vi "CPP_CalcTubingCorrection.vi"() -> (5 "Plug in titles":string[](array[string]), 7 "Plug in values":string[](array[string]))   [LabVIEW 2013]
uses:
  <vilib>/Analysis/baseanly.llb/Mean (DBL).vi
  Globals/Meas_global.vi
  <vilib>/Analysis/NI_AALBase.lvlib
  <vilib>/Analysis/NI_AALPro.lvlib
panel:
  in  "Tab Control":enum32{"TubingCorrection", "Setup"}(tab)
  in  "RefXducer":i32(ring) items=["Mano (Pref)", "Mano (P15)"]
  in  "TestXducer":i32(ring) items=["Mano (Pref)", "Mano (P15)"]
  out "Time Traces":cluster{dbl, dbl, dbl[][]}(graph)
  out "Spectra":cluster{dbl, "df (Hz)":dbl, dbl[][]}(graph)
  in  "stop":bool
  in  "Pause Button":bool
  in  "Pause(ms)":u32=500
  in  "Coherence Threshold":dbl=0.98
  out "Coefficients Smoothed and Normalized":bool
  in  "Decimate Correction File?":bool=TRUE
  in  "Smooth Correction File?":bool=TRUE
  in  "CorrectionFileDestinationPath":path
  in  "fcut (Hz)":dbl=1000.0
  in  "Cutoff type":string(combo)="Brickwall"
  out "SD(boosted)":dbl format="%.3e"
  out "SD(ref)":dbl format="%.3e"
  out "SD(Boostederror%)":dbl format="%#_3g"
  out "Current Block No":i32
  in  "LowFrequencySmoothingFloor":dbl=3.0
  in  "LowFrequencySmoothingCeiling":dbl=7.0
  in  "ExistingTubingCorrectionFile":path
  in  "Apply Phase Correction?":bool=TRUE
  in  "Save Files?":bool
  in  "Use Existing Correction File?":bool
  out "df (Hz)":dbl format="%.6f"
  in  "Decimation Term":i32=10
  out "OutputString":string
  in  "N Points To Average Either Side":i32=10
  in  "Force Phase 0 Intercept?":bool=TRUE
  out "SD(muted)":dbl format="%.3e"
  out "SD(Mutederror%)":dbl format="%#_3g"
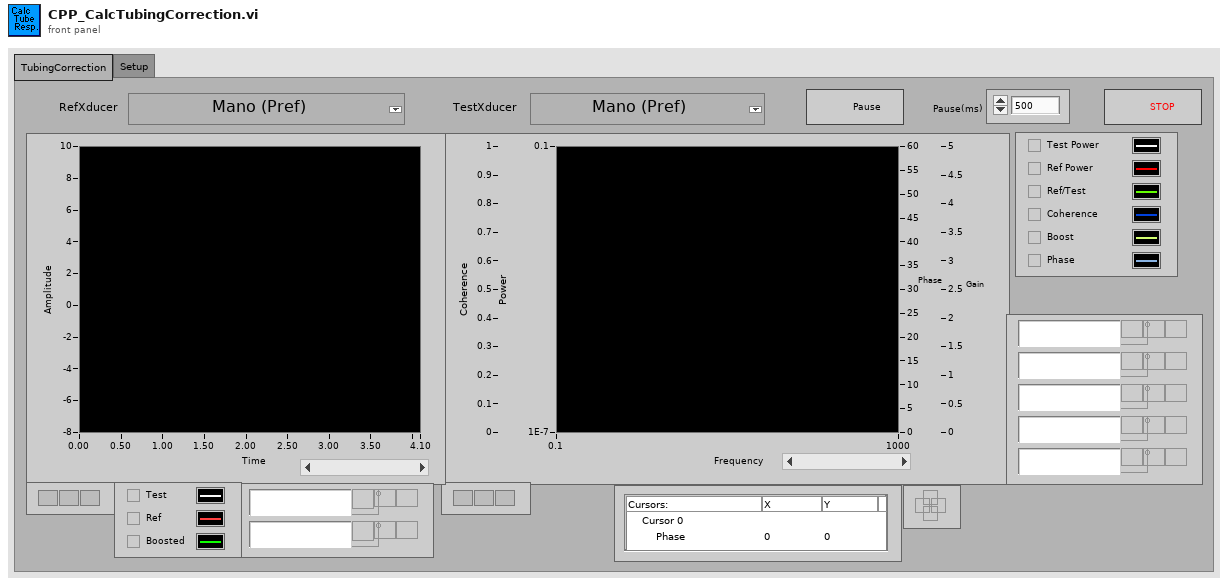
[diagram p1: front panel]
types:
  T1 = typedef "Analysis_info_cluster.ctl" = cluster{"Colour":u32, "Inst type":T2, "Inst name":string, "Symbol":string, "Code name":string, "Extra Info":string, "Inst Array":T3, "Extra Titles":string[], "Extra Values":string[], "U":dbl, "u^2":dbl, "u^3":dbl, "u^4":dbl, "Skew_u":dbl, "Kurt_u":dbl, "Sd Error in Mean":dbl, "% u'/U":dbl, "X":dbl, "Y":dbl, "Z":dbl, "Timescale integral to 25%":dbl, "Sd Error in Variance":dbl, "Calib File":path, "Calib Constants":dbl[], "Output Position":bool, "Full Stats":bool, "Av Sampling Rate":dbl, "Av No of Samples":dbl, "Total Meas Time (s)":dbl, "ADAM Ch Name":string}
  T2 = typedef "Inst_type.ctl" = enum16{"Propeller anemometer", "Raw voltage", "Pressure Transducer", "Pitot-static tube", "Preston tube", "Hot wire", "Cross wire 1", "Cross wire 2", "Generic Linear", "Generic Polynomial", "Generic BackPoly", "Fast FID", "Thermocouple", "Cold wire", "Pulsed Wire", "LDA Vel", "LDA Tran time", "LDA Arr time"}
  T3 = typedef "Instrument_Array.ctl" = enum16{"PWA", "LDA", "Analogue"}
  T4 = typedef "Time_Trace_Cluster.ctl" = cluster{"Weighting":dbl[], "Time (s)":dbl[], "Voltage":dbl[], "Eng Values":dbl[]}
  T5 = enum16{"open", "replace", "create", "open or create", "replace or create", "replace or create with confirmation"}
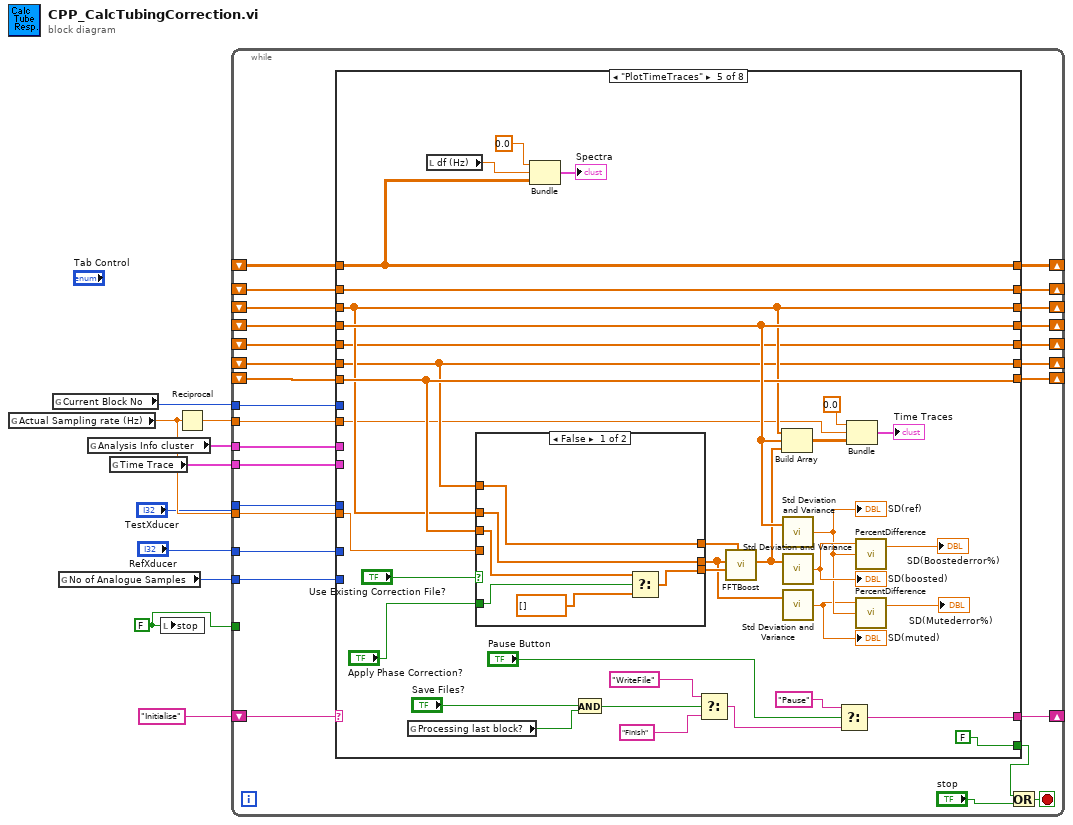
[diagram p0: block diagram]
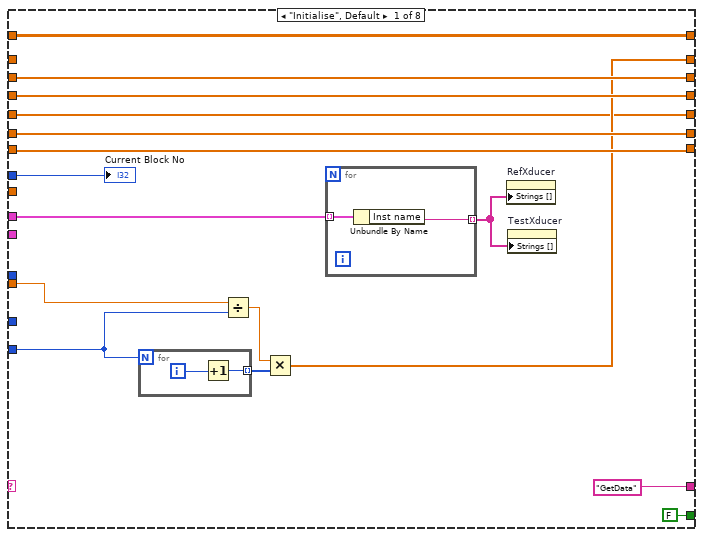
[diagram p2: hidden frame]
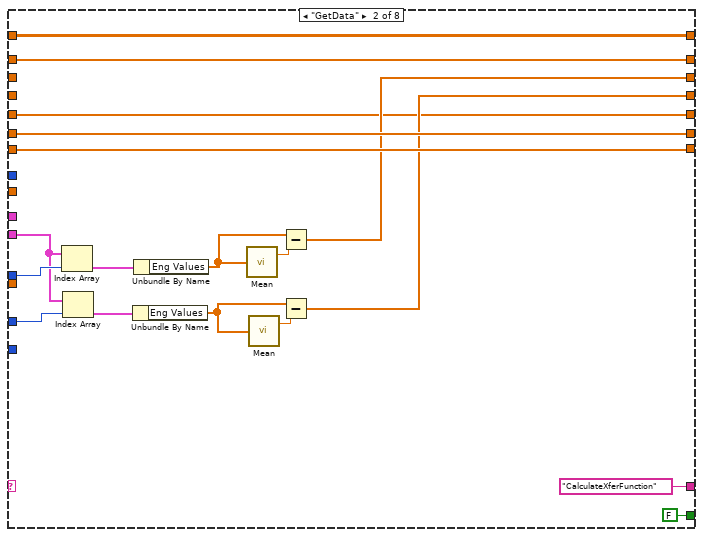
[diagram p3: hidden frame]
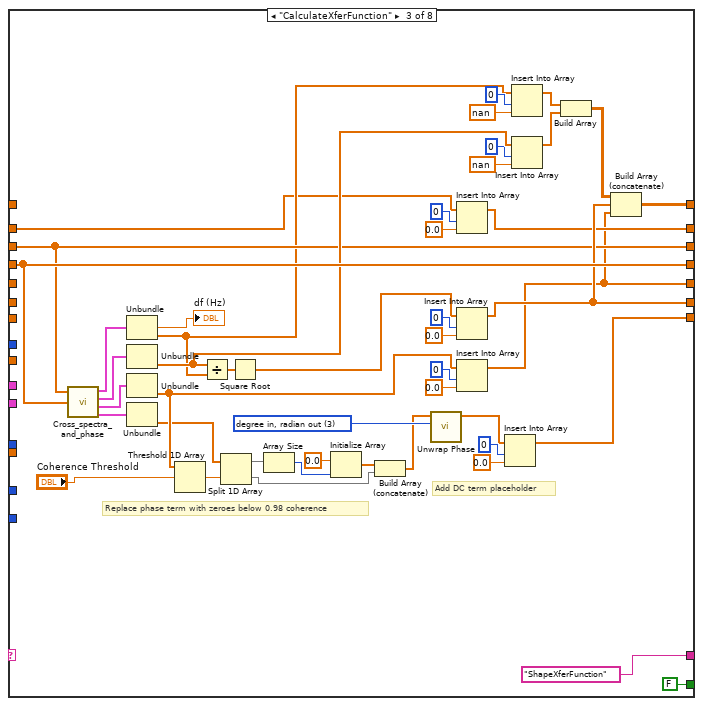
[diagram p4: hidden frame]
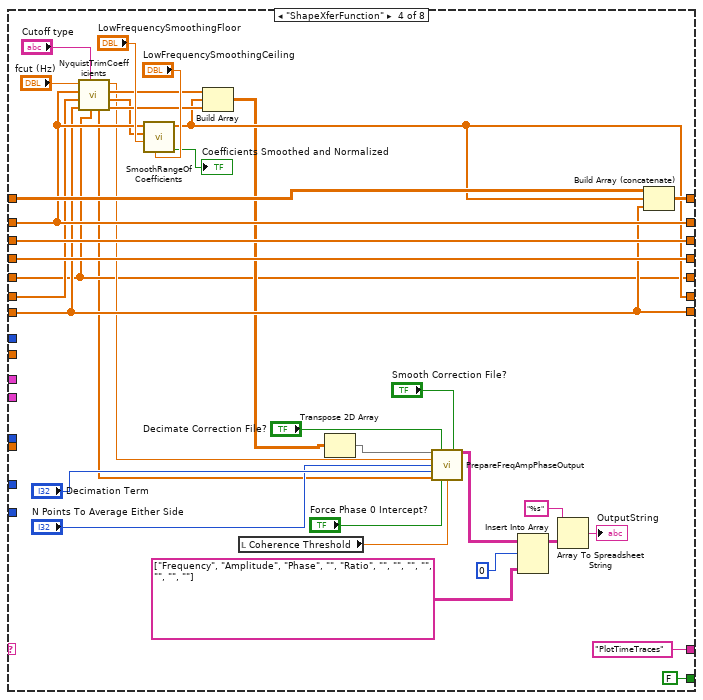
[diagram p5: hidden frame]
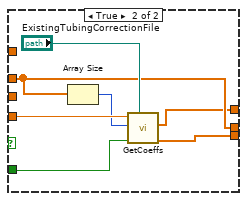
[diagram p6: hidden frame]
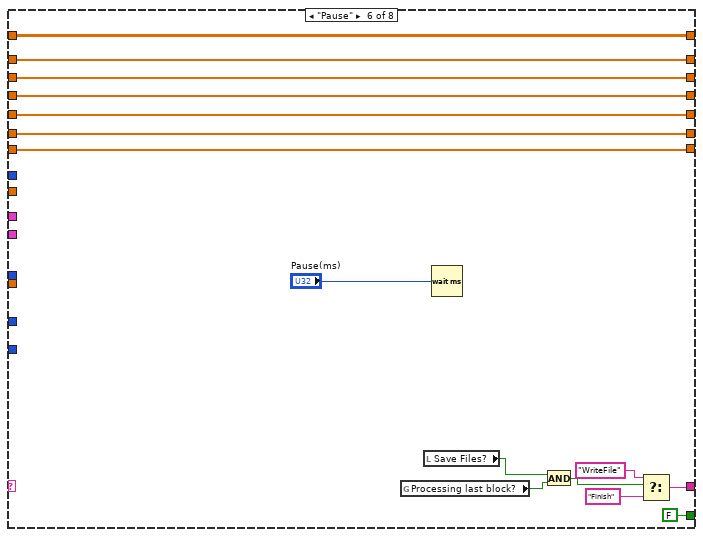
[diagram p7: hidden frame]
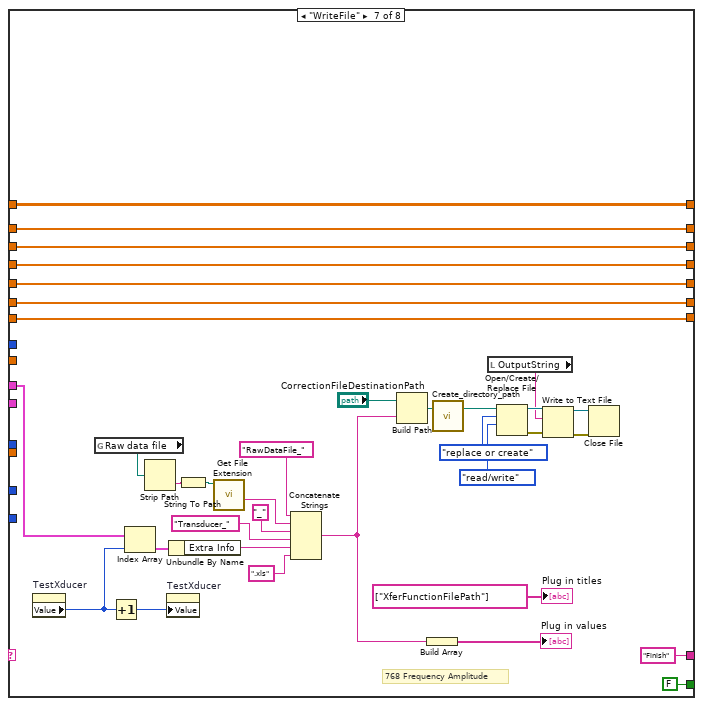
[diagram p8: hidden frame]
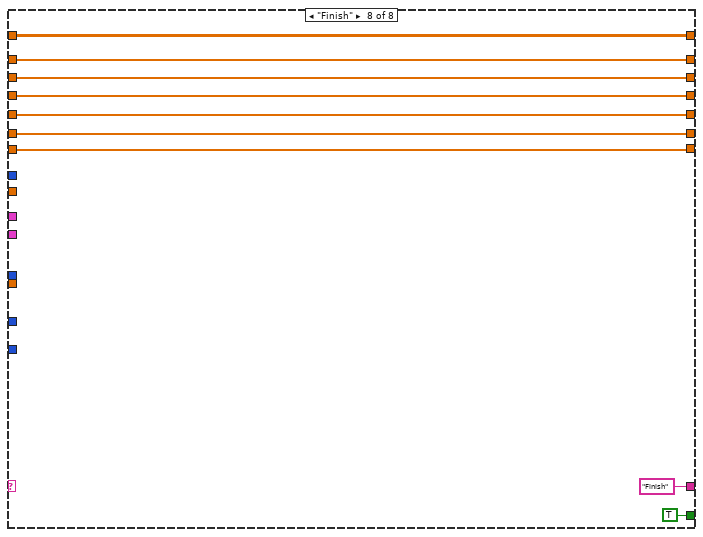
[diagram p9: hidden frame]
diagram:
  w9 = FALSE ("stop")
  n1 = global read "Meas_global.vi" "Actual Sampling rate (Hz)"() -> (w3:dbl)
  n2 = global read "Meas_global.vi" "Current Block No"() -> (w7:i32)
  n3 = global read "Meas_global.vi" "No of Analogue Samples"() -> (w2:i32)
  n4 = global read "Meas_global.vi" "Analysis Info cluster"() -> (w6:T1[])
  n5 = global read "Meas_global.vi" "Time Trace"() -> (w5:T4[])
  n6 = local write "stop"(w9) -> ()
  n7 = Reciprocal(x=w3) -> (1/x=w4:dbl)
  n8 = while {
    shift-right: [w33] -> _
    shift-left: "Initialise" -> [w37]
    tunnel: w6 -> [w36]
    tunnel: "RefXducer" -> [w34]
    tunnel: w4 -> [w32]
    tunnel: w9 -> [_]
    shift-right: [w31] -> _
    shift-left: _ -> [w29]
    shift-right: [w30] -> _
    shift-left: _ -> [w28]
    tunnel: w7 -> [w27]
    tunnel: w5 -> [w26]
    shift-right: [w25] -> _
    shift-left: _ -> [w24]
    tunnel: w3 -> [w23]
    shift-right: [w22] -> _
    shift-left: _ -> [w21]
    tunnel: w2 -> [w20]
    shift-right: [w19] -> _
    shift-left: _ -> [w18]
    shift-right: [w17] -> _
    shift-left: _ -> [w16]
    tunnel: "TestXducer" -> [w35]
    shift-right: [w12] -> _
    shift-left: _ -> [w11]
    stop <- w14 stop-if-true
    n9 = case shown="\"PlotTimeTraces\"" w37 {
      tunnel: w36 -> [w49 _ _ _ _ _ w234 _]
      tunnel: w35 -> [_ w75 _ _ _ _ _ _]
      tunnel: w34 -> [_ w74 _ _ _ _ _ _]
      tunnel: ["GetData" "CalculateXferFunction" "ShapeXferFunction" ("t") "PlotTimeTraces" ("t") w189 w210 "Finish" ("t") "Finish" ("t")] -> w33
      tunnel: w32 -> [_ _ _ _ w164 _ _ _]
      tunnel: [w52 w61 w93 w156 w180 w220 w255 w264] -> w31
      tunnel: [w51 w60 w114 w155 w182 w219 w254 w263] -> w30
      tunnel: w29 -> [w52 _ w93 w156 w180 w220 w255 w264]
      tunnel: w28 -> [w51 _ w114 w155 w182 w219 w254 w263]
      tunnel: w27 -> [w50 _ _ _ _ _ _ _]
      tunnel: w26 -> [_ w70 _ _ _ _ _ _]
      tunnel: [w47 w68 w100 w133 w178 w216 w251 w260] -> w22
      tunnel: [w48 w69 w95 w145 w181 w217 w252 w261] -> w25
      tunnel: w24 -> [w48 w69 _ w145 w181 w217 w252 w261]
      tunnel: w23 -> [w46 _ _ _ w163 _ _ _]
      tunnel: w21 -> [w47 w68 _ w146 w178 w216 w251 w260]
      tunnel: w20 -> [w45 _ _ _ _ _ _ _]
      tunnel: [w44 w67 w88 w147 w179 w215 w250 w259] -> w19
      tunnel: w18 -> [_ w67 w89 w147 w179 w215 w250 w259]
      tunnel: [w43 w66 w121 w151 w185 w214 w249 w258] -> w17
      tunnel: w16 -> [w43 w66 _ w152 w185 w214 w249 w258]
      tunnel: [FALSE FALSE FALSE FALSE FALSE FALSE FALSE TRUE] -> w13
      tunnel: [w38 w58 w77 w124 w161 w206 w221 w256] -> w12
      tunnel: w11 -> [w38 w58 _ w124 w161 w206 w221 w256]
      frame "Initialise", Default {
        n10 = for {
          N: w45 -> [_]
          tunnel: [w54] -> w41 mode=indexing
          i -> [w55]
          n11 = Increment(x=w55) -> (x+1=w54:i32)
        }
        n12 = Divide(x=w46, y=w45) -> (x/y=w40:dbl)
        n13 = Multiply(x=w40, y=w41) -> (x*y=w44:dbl[])
        n14 = for {
          tunnel: w49 -> [w57] mode=indexing
          tunnel: [w56] -> w42 mode=indexing
          n15 = Unbundle By Name(w57) -> ("Inst name"=w56:string)
        }
        n16 = property on="RefXducer" class="Ring (strict)"("Strings []"=w42) -> ()  [unwired: 2 in, 2 out]
        n17 = property on="TestXducer" class="Ring (strict)"("Strings []"=w42) -> ()  [unwired: 2 in, 2 out]
        "Current Block No" <- w50
      }
      frame "GetData" {
        n18 = Index Array(array=w70, index=w75) -> (element=w72:T4)
        n19 = Index Array(array=w70, index=w74) -> (element=w71:T4)
        n20 = Unbundle By Name(w71) -> ("Eng Values"=w62:dbl[])
        n21 = Unbundle By Name(w72) -> ("Eng Values"=w63:dbl[])
        n22 = call-poly <vilib>:"Mean.vi"("X"=w63) -> ("mean"=w64:dbl)  [unwired: 1 out]
        n23 = call-poly <vilib>:"Mean.vi"("X"=w62) -> ("mean"=w65:dbl)  [unwired: 1 out]
        n24 = Subtract(x=w63, y=w64) -> (x-y=w61:dbl[])
        n25 = Subtract(x=w62, y=w65) -> (x-y=w60:dbl[])
      }
      frame "CalculateXferFunction" {
        w116 = 3 items=["radian in, radian out", "radian in, degree out", "degree in, degree out", "degree in, radian out"] ("phase unit")
        # "Replace phase term with zeroes below 0.98 coherence"
        # "Add DC term placeholder"
        n26 = call "Cross_spectra_and_phase.vi"("U1"=w93, "U2"=w114) -> ("U1 spectra"=w120:cluster{dbl, dbl, dbl[]}, "U2 spectra"=w119:cluster{dbl, dbl, dbl[]}, "U1 U2 coherence"=w118:cluster{dbl, dbl, "Coherence array":dbl[]}, "U1 U2 phase"=w117:cluster{dbl, dbl, "Phase array":dbl[]})  [unwired: 3 out]
        n27 = Unbundle(w120) -> (→"df (Hz)":dbl, w92:dbl[])  [unwired: 1 out]
        n28 = Unbundle(w119) -> (w104:dbl[])  [unwired: 2 out]
        n29 = Unbundle(w118) -> ("Coherence array"=w87:dbl[])  [unwired: 2 out]
        n30 = Unbundle(w117) -> ("Phase array"=w85:dbl[])  [unwired: 2 out]
        n31 = Threshold 1D Array(2:"Coherence Threshold", 3:w87) -> (0:w86:dbl)  [unwired: 1 in]
        n32 = Divide(x=w104, y=w92) -> (x/y=w112:dbl[])
        n33 = Split 1D Array(array=w85, index=w86) -> (first subarray=w84:dbl[], second subarray=w83:dbl[])
        n34 = Square Root(x=w112) -> (sqrt(x)=w101:dbl[])
        n35 = Array Size(array=w84) -> (size(s)=w82:i32)
        n36 = Initialize Array(0.0 ("element"), w82) -> (w81:dbl[])
        n37 = Build Array (concatenate)(w81, w83) -> (w80:dbl[])
        n38 = call <vilib>:"Unwrap Phase.vi"("phase unit"=w116, "Phase"=w80) -> ("Unwrapped Phase"=w79:dbl[])  [unwired: 8 in, 1 out]
        n39 = Insert Into Array(array=w89, index=0, new element=0.0 ("new element/subarray")) -> (w88:dbl[])
        n40 = Insert Into Array(array=w101, index=0, new element=0.0 ("new element/subarray")) -> (w100:dbl[])
        n41 = Insert Into Array(array=w87, index=0, new element=0.0 ("new element/subarray")) -> (w77:dbl[])
        n42 = Insert Into Array(array=w79, index=0, new element=0.0 ("new element/subarray")) -> (w95:dbl[])
        n43 = Insert Into Array(array=w92, index=0, new element=nan ("new element/subarray")) -> (w106:dbl[])
        n44 = Insert Into Array(array=w104, index=0, new element=nan ("new element/subarray")) -> (w105:dbl[])
        n45 = Build Array(w106, w105) -> (w113:dbl[][])
        n46 = Build Array (concatenate)(w113, w100, w77) -> (w121:dbl[][])
      }
      frame "ShapeXferFunction" {
        n47 = call "NyquistTrimCoefficients.vi"("Coherence"=w124, "Cutoff type"="Cutoff type", "InterpolatedPhase"=w145, "InterpolatedCoefficients"=w146, "Frequencies"=w147, "fcut (Hz)"="fcut (Hz)") -> ("NyquistLimitedPhase"=w137:dbl[], "NyquistLimitedCoefficients"=w136:dbl[], "NyquistLimitedFrequency"=w135:dbl[], "fcut Index"=w132:dbl, "NyquistLimitedCoherence"=w123:dbl[])  [unwired: 1 in]
        n48 = call "SmoothRangeOfCoefficients.vi"("LFSmoothingCeiling"="LowFrequencySmoothingCeiling", "LFSmoothingFloor"="LowFrequencySmoothingFloor", "NyquistLimitedCoefficients In"=w136, "Frequencies In"=w147) -> ("Coefficients Smoothed and Normalized"=→"Coefficients Smoothed and Normalized":bool, "NyquistLimitedCoefficients Out"=w133:dbl[])  [unwired: 5 in, 1 out]
        n49 = Build Array(w135, w133, w137) -> (w129:dbl[][])
        n50 = local read "Coherence Threshold"() -> (w122:dbl)
        n51 = Transpose 2D Array(2D array=w129) -> (transposed array=w128:dbl[][])
        n52 = call "PrepareFreqAmpPhaseOutput.vi"("Array in"=w128, "Decimate Correction File?"="Decimate Correction File?", "Smooth Correction File?"="Smooth Correction File?", "fcut Index"=w132, "N Points To Average Either Side"="N Points To Average Either Side", "Decimation Term"="Decimation Term", "Coherence"=w123, "Force Phase 0 Intercept?"="Force Phase 0 Intercept?", "Coherence Threshold"=w122) -> ("Array out"=w139:string[][])  [unwired: 6 in]
        n53 = Insert Into Array(array=w139, index (row)=0, new element=string[][] [["Frequency", "Amplitude", "Phase"], ["", "Ratio", ""], ["", "", ""], ["", "", ""]]) -> (w141:string[][])  [unwired: 1 in]
        n54 = Array To Spreadsheet String(array=w141, 3:"%s" ("format string")) -> (spreadsheet string=→"OutputString":string)  [unwired: 1 in]
        n55 = Build Array (concatenate)(w152, w133, w145) -> (w151:dbl[][])
      }
      frame "PlotTimeTraces" {
        n56 = global read "Meas_global.vi" "Processing last block?"() -> (w172:bool)
        n57 = local read "df (Hz)"() -> (w168:dbl)
        n58 = case shown="False" "Use Existing Correction File?" {
          tunnel: w181 -> [w195 _]
          tunnel: w180 -> [w198 w202]
          tunnel: w178 -> [w197 _]
          tunnel: w163 -> [_ w204]
          tunnel: [w197 w201] -> w167
          tunnel: [w198 w202] -> w160
          tunnel: [w193 w200] -> w166
          tunnel: "Apply Phase Correction?" -> [w196 w199]
          frame False {
            n59 = Select(t=w195, s=w196, f=dbl[] [] ("NyquistLimitedPhase")) -> (s? t:f=w193:dbl[])
          }
          frame True {
            n60 = Array Size(array=w202) -> (size(s)=w203:i32)
            n61 = call "GetCoeffs.vi"("PathToFile"="ExistingTubingCorrectionFile", "Apply Phase Correction?"=w199, "SignalLength"=w203, "fs (Hz)"=w204) -> ("NyquistLimitedPhase"=w200:dbl[], "NyquistLimitedCoefficients"=w201:dbl[])  [unwired: 6 in]
          }
        }
        n62 = Bundle(0.0, "df (Hz)"=w168, w185) -> (→"Spectra":cluster{dbl, "df (Hz)":dbl, dbl[][]})  [unwired: 1 in]
        n63 = And(x="Save Files?", y=w172) -> (x .and. y?=w171:bool)
        n64 = Select(t="WriteFile", s=w171, f="Finish") -> (s? t:f=w175:string)
        n65 = call "FFTBoost.vi"("CompensationCoefficients"=w167, "PhaseCorrection"=w166, "mutedData"=w160) -> ("boostedData"=w165:dbl[])  [unwired: 1 in, 7 out]
        n66 = Build Array(w180, w182, w165) -> (w188:dbl[][])
        n67 = call <vilib>:"Std Deviation and Variance.vi"("X"=w182) -> ("standard deviation"=w159:dbl)  [unwired: 1 in, 2 out]
        "SD(ref)" <- w159
        n68 = call <vilib>:"Std Deviation and Variance.vi"("X"=w165) -> ("standard deviation"=w183:dbl)  [unwired: 1 in, 2 out]
        "SD(boosted)" <- w183
        n69 = call <vilib>:"Std Deviation and Variance.vi"("X"=w160) -> ("standard deviation"=w158:dbl)  [unwired: 1 in, 2 out]
        "SD(muted)" <- w158
        n70 = Select(t="Pause", s="Pause Button", f=w175) -> (s? t:f=w189:string)
        n71 = Bundle(0.0, w164, w188) -> (→"Time Traces":cluster{dbl, dbl, dbl[][]})  [unwired: 1 in]
        n72 = call "PercentDifference.vi"("Basis"=w159, "Comparee"=w183) -> ("PercentageDifference"=→"SD(Boostederror%)":dbl)  [unwired: 1 in, 1 out]
        n73 = call "PercentDifference.vi"("Basis"=w159, "Comparee"=w158) -> ("PercentageDifference"=→"SD(Mutederror%)":dbl)  [unwired: 1 in, 1 out]
      }
      frame "Pause" {
        n74 = global read "Meas_global.vi" "Processing last block?"() -> (w208:bool)
        n75 = local read "Save Files?"() -> (w209:bool)
        n76 = Wait (ms)(milliseconds to wait="Pause(ms)") -> ()  [unwired: 1 out]
        n77 = And(x=w209, y=w208) -> (x .and. y?=w207:bool)
        n78 = Select(t="WriteFile", s=w207, f="Finish") -> (s? t:f=w210:string)
      }
      frame "WriteFile" {
        # "768 Frequency Amplitude"
        n79 = property on="TestXducer" class="Ring (strict)"() -> ("Value"=w223:i32)  [unwired: 2 in, 2 out]
        n80 = global read "Meas_global.vi" "Raw data file"() -> (w228:path)
        n81 = Increment(x=w223) -> (x+1=w224:i32)
        n82 = Index Array(array=w234, index=w223) -> (element=w233:T1)
        n83 = Strip Path(path=w228) -> (name=w226:string)  [unwired: 1 out]
        n84 = property on="TestXducer" class="Ring (strict)"("Value"=w224) -> ()  [unwired: 2 in, 2 out]
        n85 = Unbundle By Name(w233) -> ("Extra Info"=w230:string)
        n86 = String To Path(string=w226) -> (path=w225:path)
        n87 = call <vilib>:"Get File Extension.vi"("file"=w225) -> ("filename without extension"=w227:string)  [unwired: 7 in, 3 out]
        n88 = Concatenate Strings("RawDataFile_" ("string"), w227, "_" ("string"), "Transducer_" ("string"), w230, ".xls" ("string")) -> (w244:string)
        n89 = Build Path(base path="CorrectionFileDestinationPath", name or relative path=w244) -> (appended path=w236:path)
        n90 = Build Array(w244) -> (→"Plug in values":string[])
        n91 = call "Create_directory_path.vi"("Path name"=w236) -> ("Path name Out"=w235:path)  [unwired: 1 in, 1 out]
        n92 = local read "OutputString"() -> (w239:string)
        n93 = Open/Create/Replace File(file path (use dialog)=w235, operation (0:open)=T5."replace or create", access (0:read/write)=enum16{"read/write", "read-only", "write-only"}."read/write") -> (refnum out=w240:refnum<file>, error out=w241:errorcluster)  [unwired: 3 in, 1 out]
        n94 = Write to Text File(file (use dialog)=w240, text=w239, error in=w241) -> (refnum out=w237:refnum<file>, error out=w238:errorcluster)  [unwired: 1 in, 1 out]
        n95 = Close File(refnum=w237, error in=w238) -> ()  [unwired: 2 out]
        "Plug in titles" <- string[] ["XferFunctionFilePath"] ("Add in values")
      }
      frame "Finish" {
      }
    }
    n96 = Or(x=w13, y="stop") -> (x .or. y?=w14:bool)
  }
